vi "SubVI_EXA Binary 2 file.vi"(2 "error in (no error)":errorcluster, 3 "Path":path, 4 "VISA resource in":refnum<visa-resource-name>) -> (0 "error out":errorcluster, 1 "VISA resource out":refnum<visa-resource-name>)   [LabVIEW 2016]
doc: "read binary block to a file"
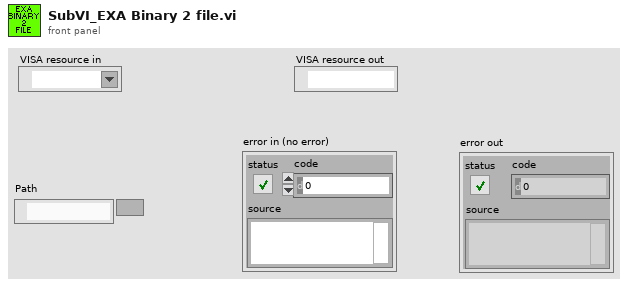
[diagram p1: front panel]
types:
  T1 = enum16{"big-endian, network order", "native, host order", "little-endian"}
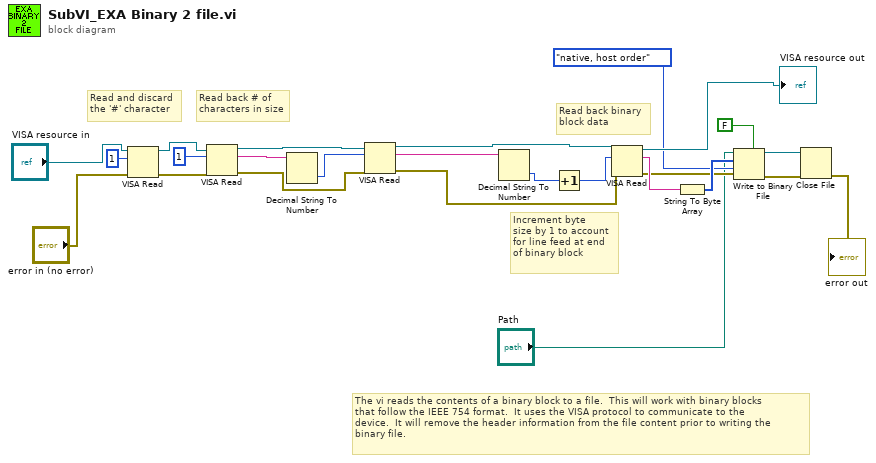
[diagram p0: block diagram]
diagram:
  # "The vi reads the contents of a binary block to a file.  This will work with binary blocks\nthat follow the IEEE 754 format.  It uses the VISA protocol to communicate to the\ndevice.  It will remove the header information from the file content prior to writing the\nbinary file."
  # "Increment byte\nsize by 1 to account\nfor line feed at end\nof binary block"
  # "Read back binary\nblock data"
  # "Read back # of\ncharacters in size"
  # "Read and discard\nthe '#' character"
  n1 = VISA Read(VISA resource name="VISA resource in", byte count=u32 1, error in (no error)="error in (no error)") -> (VISA resource name out=w15:refnum<visa-resource-name>, error out=w11:errorcluster)  [unwired: 2 out]
  n2 = VISA Read(VISA resource name=w15, byte count=u32 1, error in (no error)=w11) -> (VISA resource name out=w14:refnum<visa-resource-name>, read buffer=w23:string, error out=w10:errorcluster)  [unwired: 1 out]
  n3 = Decimal String To Number(string=w23) -> (number=w22:i32)  [unwired: 2 in, 1 out]
  n4 = VISA Read(VISA resource name=w14, byte count=w22, error in (no error)=w10) -> (VISA resource name out=w13:refnum<visa-resource-name>, read buffer=w21:string, error out=w9:errorcluster)  [unwired: 1 out]
  n5 = Decimal String To Number(string=w21) -> (number=w20:i32)  [unwired: 2 in, 1 out]
  n6 = Increment(x=w20) -> (x+1=w19:i32)
  n7 = VISA Read(VISA resource name=w13, byte count=w19, error in (no error)=w9) -> (VISA resource name out=→"VISA resource out":refnum<visa-resource-name>, read buffer=w18:string, error out=w8:errorcluster)  [unwired: 1 out]
  n8 = String To Byte Array(string=w18) -> (unsigned byte array=w17:u8[])
  n9 = Write to Binary File(file (use dialog)="Path", data=w17, error in=w8, 5:FALSE ("prepend array or string size? (T)"), 9:T1."native, host order" ("byte order (0:big-endian, network order)")) -> (refnum out=w4:refnum<file>, error out=w7:errorcluster)  [unwired: 1 in, 1 out]
  n10 = Close File(refnum=w4, error in=w7) -> (error out=→"error out":errorcluster)  [unwired: 1 out]
